vi "readcommand(sub).vi"(3 "errorin":errorcluster, 4 "readdelay":u32=500, 5 "Command":dbl, 6 "resourcein":refnum<visa-resource-name>) -> (0 "errorout":errorcluster, 1 "readstring":string, 2 "resourceout":refnum<visa-resource-name>)   [LabVIEW 2015]
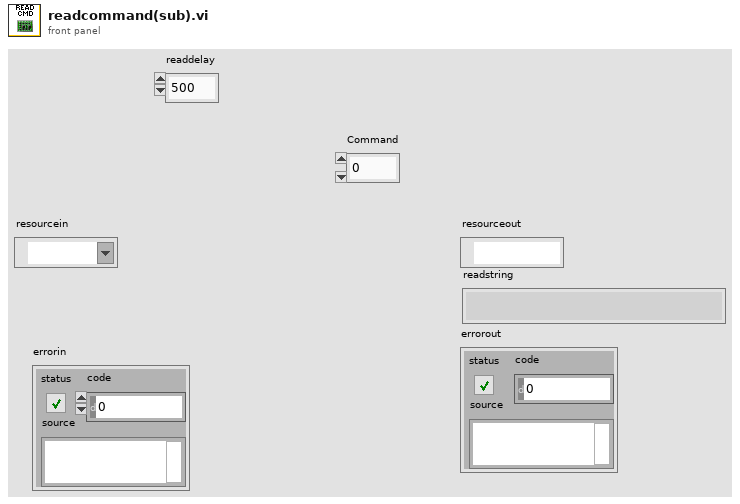
[diagram p1: front panel]
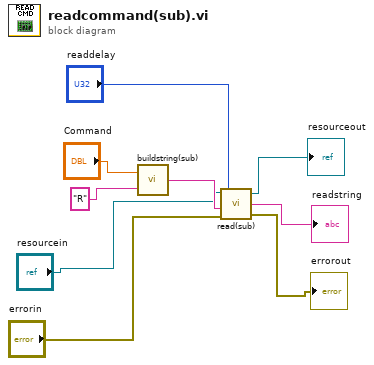
[diagram p0: block diagram]
diagram:
  n1 = call "buildstring(sub).vi"("Prefix"="R", "Command"="Command") -> ("Commandstring"=w7:string)
  n2 = call "read(sub).vi"("errorin"="errorin", "writestring"=w7, "readdelay"="readdelay", "resourcein"="resourcein") -> ("errorout"=→"errorout":errorcluster, "readstring"=→"readstring":string, "resourceout"=→"resourceout":refnum<visa-resource-name>)
